vi "十进制同步加法计数器74HC162的功能测试.vi"(0 "EP":bool, 1 "D2":bool, 2 "D3":bool, 5 "ET":bool, 7 "cp":bool, 9 "CR`":bool, 11 "LD`":bool, 12 "D1":bool, 13 "D0":bool) -> (4 "Q3":bool, 6 "Q2":bool, 8 "Q1":bool, 10 "Q0":bool, 15 "RCO":bool)   [LabVIEW 2018]
panel:
  in  "结束":bool
  # "74HC162：十进制同步加法器"
  # "CR`：异步清零端\nEP：计数使能\nLD`：数据加载\nRC0：进位输出\nET：计数控制端"
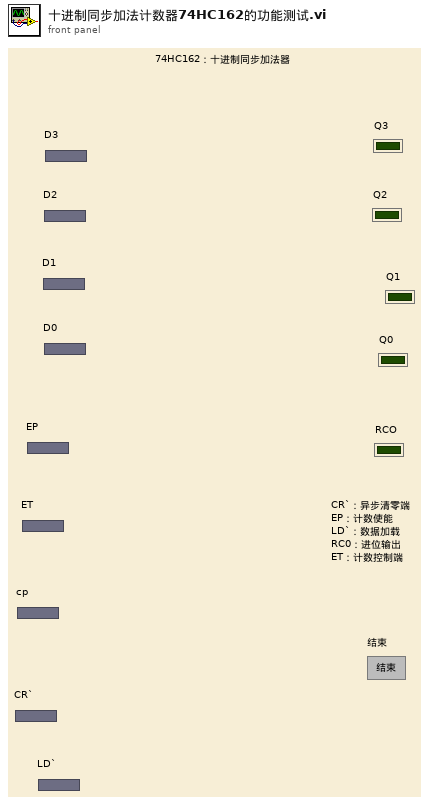
[diagram p1: front panel]
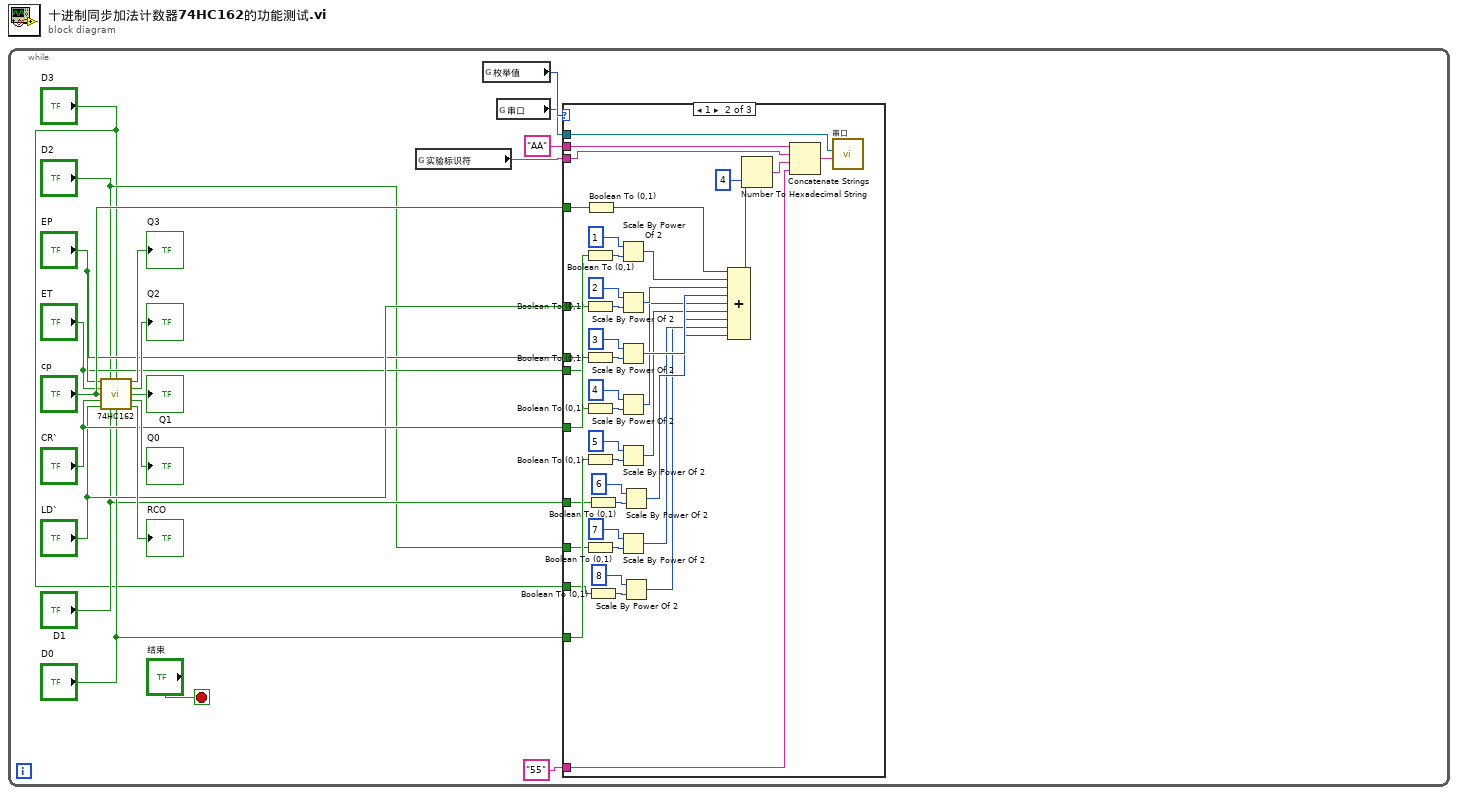
[diagram p0: block diagram]
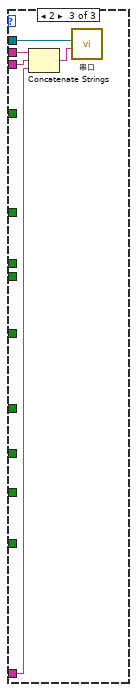
[diagram p3: hidden frame]
diagram:
  n1 = while {
    stop <- "结束" stop-if-true
    n2 = call "74HC162.vi"("EP"="EP", "D2"="D2", "D3"="D3", "ET"="ET", "cp"="cp", "CR`"="CR`", "LD`"="LD`", "D1"="D1", "D0"="D0") -> ("Q3"=→"Q3":bool, "Q2"=→"Q2":bool, "Q1"=→"Q1":bool, "Q0"=→"Q0":bool, "RCO"=→"RCO":bool)  [unwired: 2 in]
    n3 = global read "全局变量.vi" "实验标识符"() -> (w12:string)
    n4 = global read "全局变量.vi" "枚举值"() -> (w14:i8)
    n5 = global read "全局变量.vi" "串口"() -> (w13:refnum<visa-resource-name>)
    n6 = case shown="1" w14 {
      tunnel: w13 -> [_ w57 w65]
      tunnel: w12 -> [_ w56 w66]
      tunnel: "55" -> [_ w55 w63]
      tunnel: "AA" -> [_ w54 w64]
      tunnel: "cp" -> [_ w29 _]
      tunnel: "CR`" -> [_ w28 _]
      tunnel: "LD`" -> [_ w27 _]
      tunnel: "EP" -> [_ w26 _]
      tunnel: "ET" -> [_ w25 _]
      tunnel: "D0" -> [_ w24 _]
      tunnel: "D1" -> [_ w23 _]
      tunnel: "D2" -> [_ w22 _]
      tunnel: "D3" -> [_ w21 _]
      frame 0, Default {
      }
      frame 1 {
        n7 = Boolean To (0,1)(Boolean=w28) -> (0, 1=w59:i16)
        n8 = Boolean To (0,1)(Boolean=w27) -> (0, 1=w49:i16)
        n9 = Boolean To (0,1)(Boolean=w26) -> (0, 1=w47:i16)
        n10 = Boolean To (0,1)(Boolean=w25) -> (0, 1=w45:i16)
        n11 = Boolean To (0,1)(Boolean=w24) -> (0, 1=w43:i16)
        n12 = Boolean To (0,1)(Boolean=w22) -> (0, 1=w36:i16)
        n13 = Boolean To (0,1)(Boolean=w29) -> (0, 1=w61:i16)
        n14 = Boolean To (0,1)(Boolean=w23) -> (0, 1=w38:i16)
        n15 = Boolean To (0,1)(Boolean=w21) -> (0, 1=w34:i16)
        n16 = Scale By Power Of 2(n=1, x=w59) -> (x*2^n=w60:i16)
        n17 = Scale By Power Of 2(n=2, x=w49) -> (x*2^n=w50:i16)
        n18 = Scale By Power Of 2(n=3, x=w47) -> (x*2^n=w41:i16)
        n19 = Scale By Power Of 2(n=4, x=w45) -> (x*2^n=w40:i16)
        n20 = Scale By Power Of 2(n=5, x=w43) -> (x*2^n=w39:i16)
        n21 = Scale By Power Of 2(n=7, x=w36) -> (x*2^n=w31:i16)
        n22 = Scale By Power Of 2(n=6, x=w38) -> (x*2^n=w32:i16)
        n23 = Scale By Power Of 2(n=8, x=w34) -> (x*2^n=w30:i16)
        n24 = Compound Arithmetic op=ADD ("复合运算")(w61, w60, w50, w41, w40, w39, w32, w31, w30) -> (w53:i16)
        n25 = Number To Hexadecimal String(1:4, 2:w53) -> (0:w51:string)
        n26 = Concatenate Strings(w54, w56, w51, w55) -> (w62:string)
        n27 = call "串口.vi"("字符串"=w62, "VISA resource name"=w57) -> ()  [unwired: 10 in]
      }
      frame 2 {
        n28 = Concatenate Strings(w64, w66, w63) -> (w67:string)
        n29 = call "串口.vi"("字符串"=w67, "VISA resource name"=w65) -> ()  [unwired: 10 in]
      }
    }
  }
